vi "TraceLoggerTracePointListRequest_Parse.vi"(8 "error in (no error)":errorcluster, 11 "Message":T4) -> (0 "error out":errorcluster, 2 "Header":T2, 3 "TraceLoggerTracePointListRequest":T1)   [LabVIEW 2017]
uses:
  <vilib>/addons/InsightCM/MessageBus/Base/controls/Message.ctl
  <vilib>/addons/InsightCM/MessageBus/Base/controls/MessageHeader.ctl
  <vilib>/addons/InsightCM/MessageBus/Base/controls/KeyValuePair.ctl
  <vilib>/addons/InsightCM/MessageBus/MessageLibrary/TraceLogger/controls/TraceLoggerTracePointListRequest.ctl
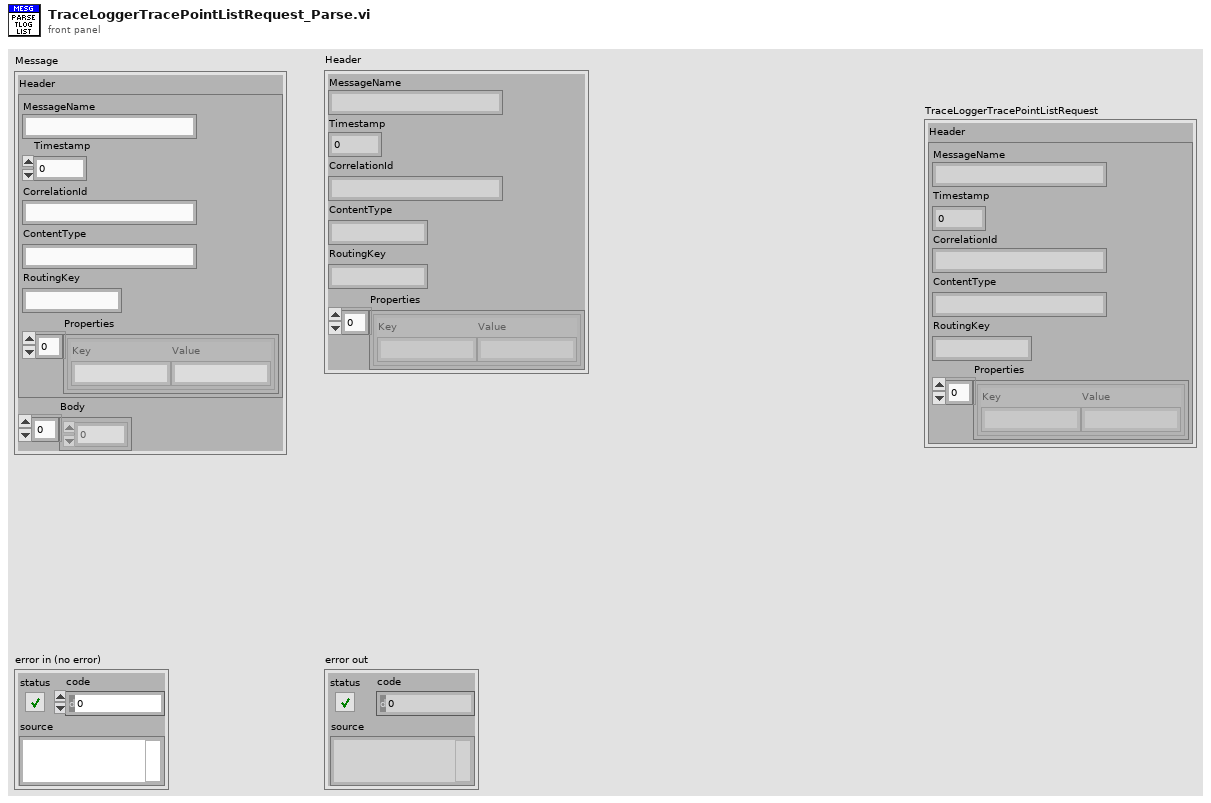
[diagram p1: front panel]
types:
  T1 = typedef "TraceLoggerTracePointListRequest.ctl" = cluster{"Header":T2}
  T2 = typedef "MessageHeader.ctl" = cluster{"MessageName":string, "Timestamp":i64, "CorrelationId":string, "ContentType":string, "RoutingKey":string, "Properties":T3[]}
  T3 = typedef "KeyValuePair.ctl" = cluster{"Key":string, "Value":string}
  T4 = typedef "Message.ctl" = cluster{"Header":T2, "Body":u8[]}
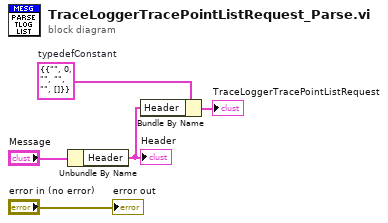
[diagram p0: block diagram]
diagram:
  w2 = T1 {"Header"={"MessageName"="", "Timestamp"=0, "CorrelationId"="", "ContentType"="", "RoutingKey"="", "Properties"=[]}}  # typedefConstant
  n1 = Unbundle By Name("Message") -> ("Header"=w4:T2)
  "Header" <- w4
  n2 = Bundle By Name(cluster=w2, "Header"=w4) -> (→"TraceLoggerTracePointListRequest":T1)
  "error out" <- "error in (no error)"
